vi "MarkerTactic.vi"(8 "error in (no error)":errorcluster, 9 "Game in":refnum<class "Game.lvclass">, 10 "Robot":refnum<class "Robot.lvclass">, 11 "MarkerTactic in":refnum<class "MarkerTactic.lvclass">) -> (0 "error out":errorcluster, 2 "Robot out":refnum<class "Robot.lvclass">, 3 "MarkerTactic out":refnum<class "MarkerTactic.lvclass">)   [LabVIEW 2023, in "MarkerTactic.lvclass"]
uses:
  MarkerTactic.lvclass
  Robot_class/Robot.lvclass
  Game_class/Game.lvclass
  Robot_class/tactics.ctl
  MarkerTacticStates.ctl
  Tactic_class/Tactic.lvclass/Tactic.ctl
  Game_class/Game.lvclass/Game.ctl
  Parameters_class/Parameters.lvclass/Parameters.ctl
  Skillbook_class/Skillbook.lvclass/Skillbook.ctl
  Robot_class/Robot.lvclass/Robot.ctl
  Skillbook_class/Read MarkerSkill.lvclass.vi
  Skillbook_class/Read FollowAttackerSkill.lvclass.vi
  Game_class/Read Parameters.lvclass.vi
  Parameters_class/Read Type of Marker.vi
  Parameters_class/Read DistanceStop.vi
  Tactic_class/Read Skillbook.vi
  Robot_class/Write tactic.vi
  Parameters_class/Parameters.lvclass
  Skillbook_class/Skillbook.lvclass
  MarkerSkill_class/MarkerSkill.lvclass
  FollowAttackerSkill_class/FollowAttackerSkill.lvclass
panel:
  out "x .or. y?":bool
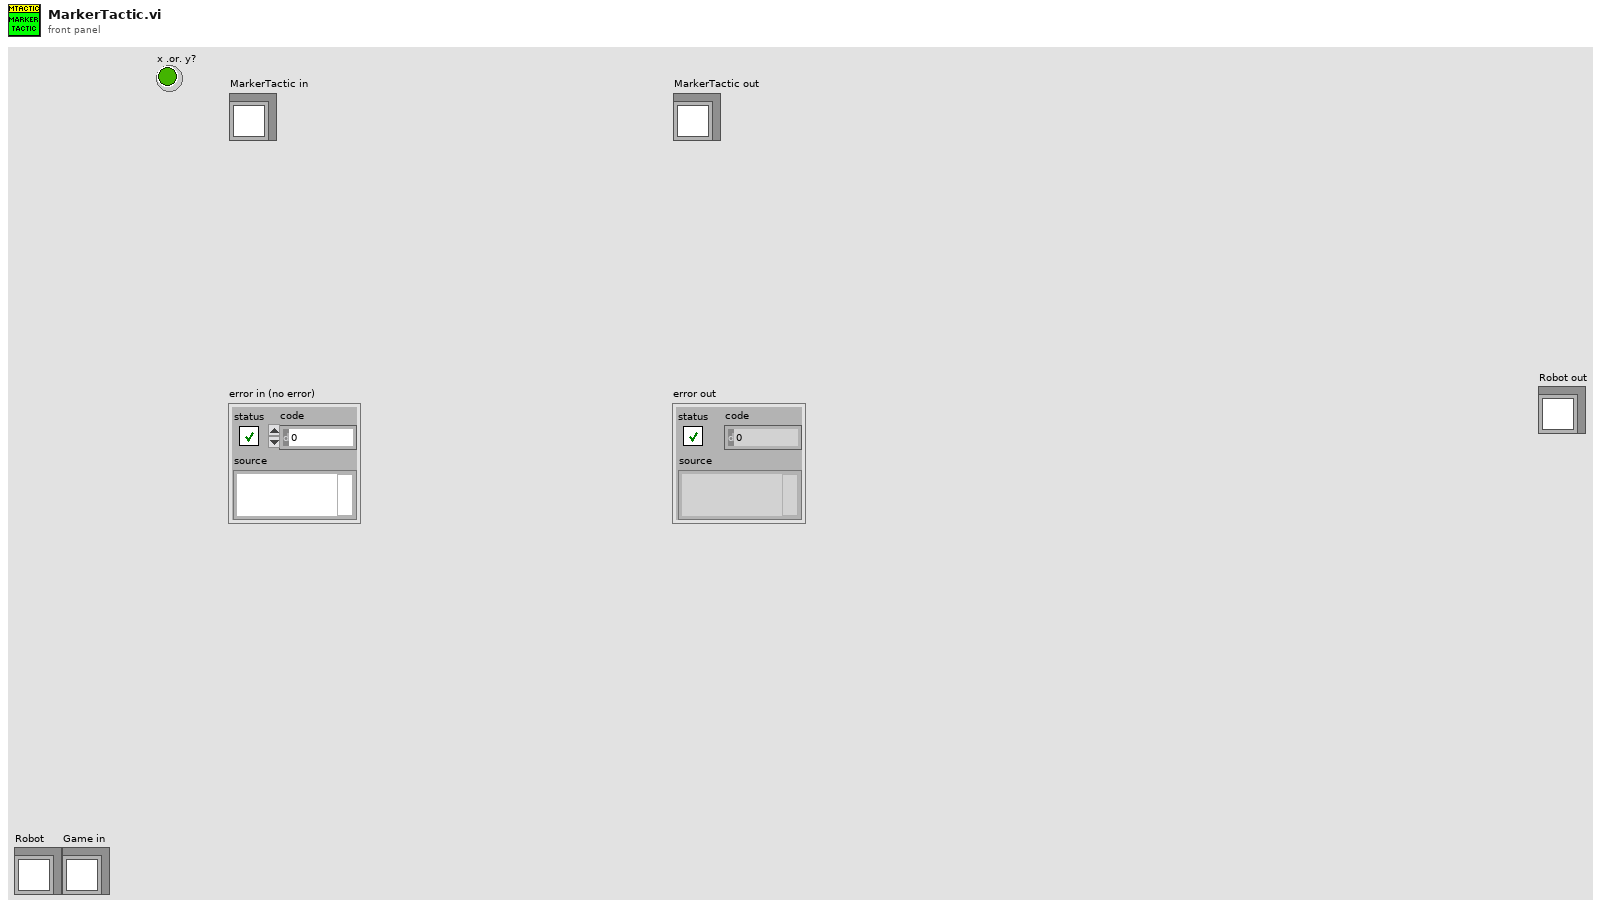
[diagram p1: front panel]
types:
  T1 = typedef "MarkerTacticStates.ctl" = enum16{"Exit", "BlockOurGoal", "FollowAttacker", "BlockEnemyPass"}
  T2 = typedef "tactics.ctl" = enum16{"ReceivePassInFuturePoint", "Roller", "PrepareRollToPassRollerGoTo", "PrepareRollToPassReceiverGoTo", "WaitRoll", "PositionToRoll", "PenaltyAttacker", "PassObserver", "PenaltyDefense", "TableReceiverTactic", "Test", "DefendGoal", "Marker", "FollowAttacker", "DefendArea", "Shoot", "AttackerAimGoal", "AttackerBallOutOfField", "AttackerBlock", "AttackerStop", "Duelist", "Halt", "ZigZag", "GoTo", "Timeout", "KickToPassReceiver", "PositionToReceivePass", "DefendAreaVSS", "DefendGoalVSS", "KickVSS", "AttackVSS", "DispBallVSS", "PenaltyAttackVSS", "WaitPass"}
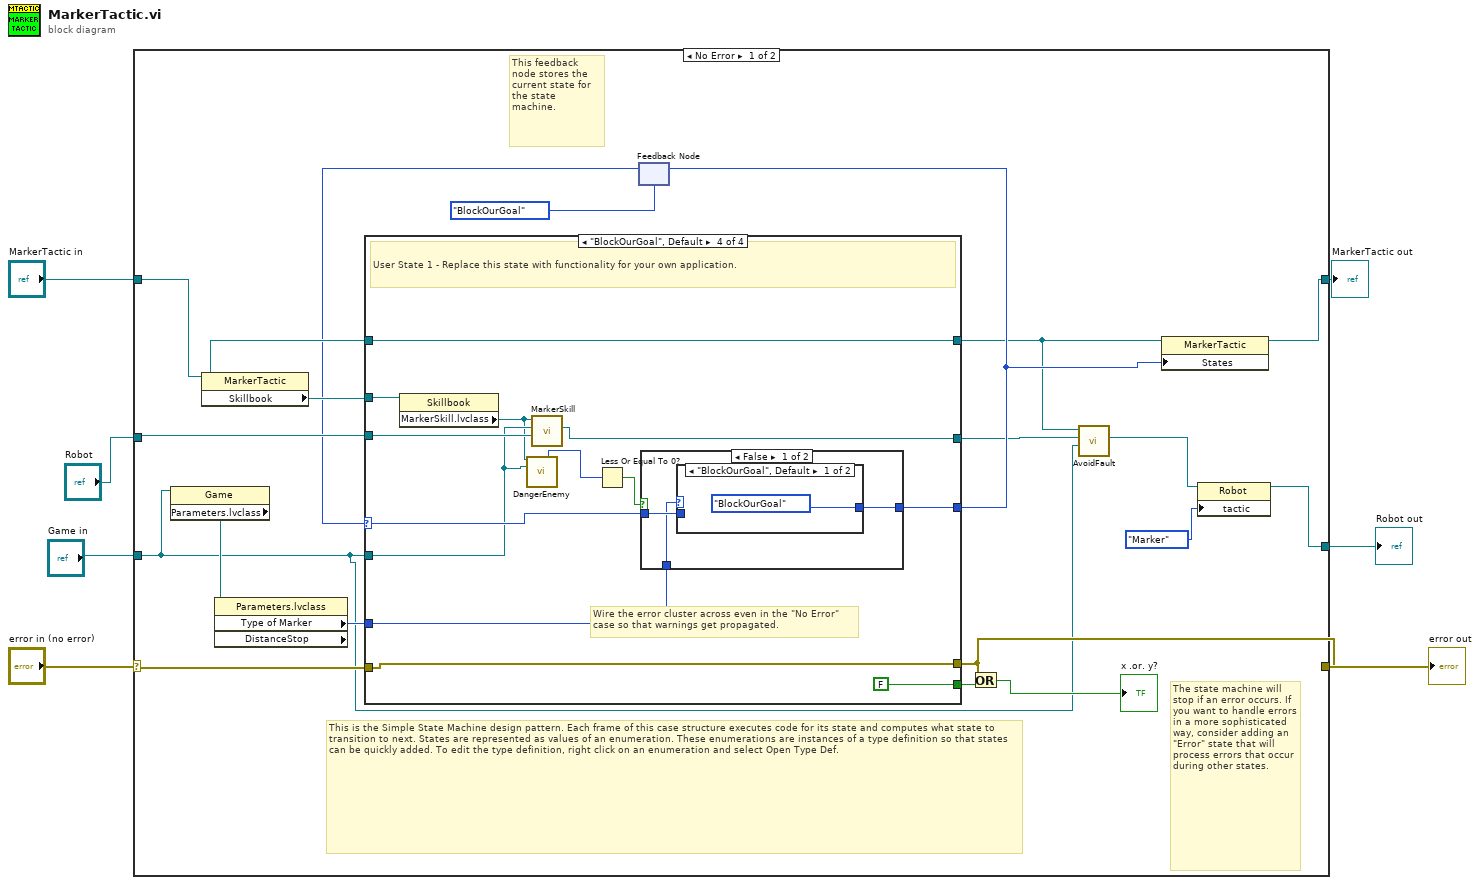
[diagram p0: block diagram]
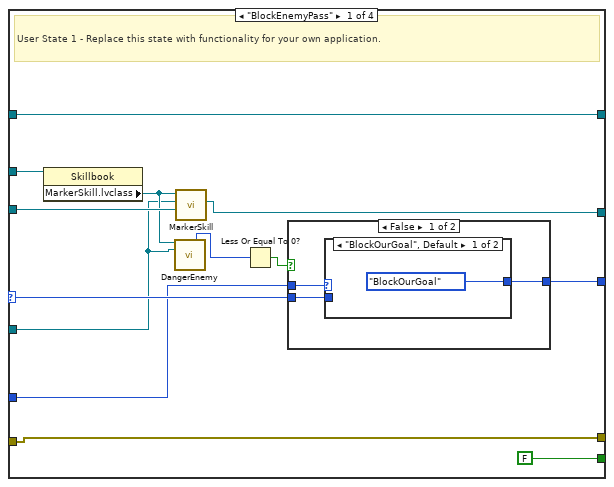
[diagram p2: hidden frame]
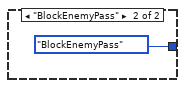
[diagram p3: hidden frame]
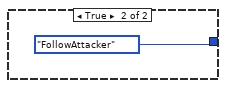
[diagram p4: hidden frame]
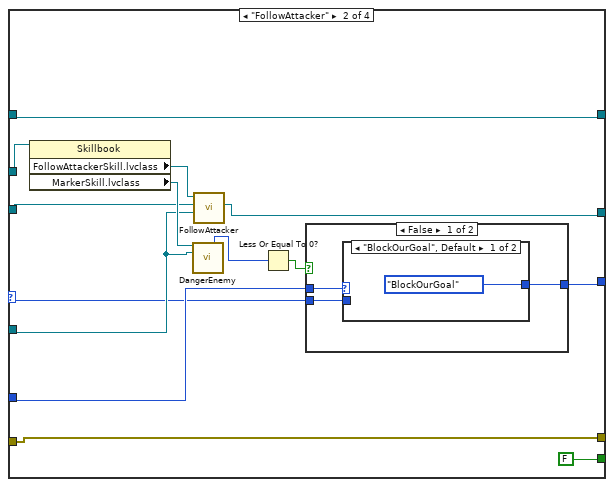
[diagram p5: hidden frame]
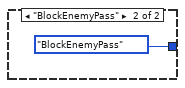
[diagram p6: hidden frame]
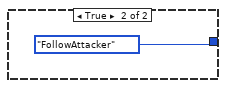
[diagram p7: hidden frame]
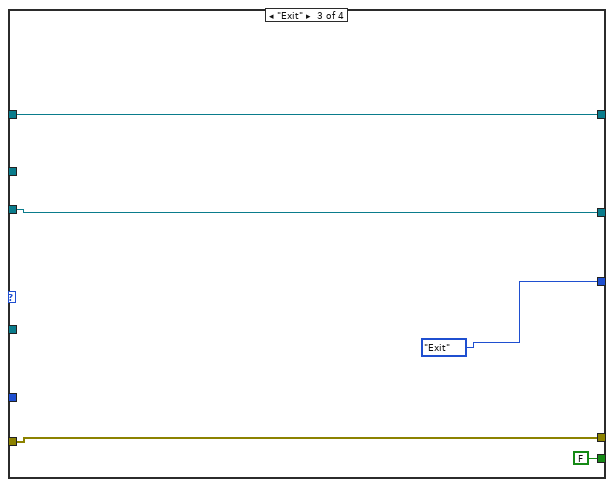
[diagram p8: hidden frame]
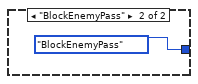
[diagram p9: hidden frame]
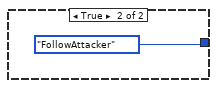
[diagram p10: hidden frame]
diagram:
  n1 = case shown="No Error" "error in (no error)" {
    selector: "error in (no error)" -> [w22 w92]
    tunnel: [w21 w92] -> w6
    tunnel: [w19 w91] -> w4
    tunnel: "MarkerTactic in" -> [w20 w91]
    tunnel: "Robot" -> [w23 w90]
    tunnel: "Game in" -> [w8 _]
    tunnel: [w14 w90] -> w1
    frame No Error {
      # "The state machine will stop if an error occurs. If you want to handle errors in a more sophisticated way, consider adding an \"Error\" state that will process errors that occur during other states."
      # "This feedback node stores the current state for the state machine."
      # "This is the Simple State Machine design pattern. Each frame of this case structure executes code for its state and computes what state to transition to next. States are represented as values of an enumeration. These enumerations are instances of a type definition so that states can be quickly added. To edit the type definition, right click on an enumeration and select Open Type Def."
      # "Wire the error cluster across even in the \"No Error\"\ncase so that warnings get propagated."
      n2 = property class="Game"(reference=w8) -> ("Parameters.lvclass"=w18:refnum<class "Parameters.lvclass">)  [unwired: 1 in, 2 out]
      n3 = property class="MarkerTactic"(reference=w20) -> ("Skillbook"=w24:refnum<class "Skillbook.lvclass">)  [unwired: 1 in, 2 out]
      n4 = property class="Parameters.lvclass" props=["Type of Marker", "DistanceStop"](reference=w18) -> ("Type of Marker"=w17:enum16{"BlockEnemyPass", "BlockOurGoal"})  [unwired: 1 in, 3 out]
      n5 = feedback #1(MarkerTacticStates."BlockOurGoal" ("States")) -> (w16:T1)
      n6 = case shown="\"BlockOurGoal\", Default" w16 {
        selector: w16 -> [w32 w49 _ w76]
        tunnel: [FALSE ("Stop Loop?") FALSE ("Stop Loop?") FALSE ("Stop Loop?") FALSE ("Stop Loop?")] -> w26
        tunnel: w24 -> [w38 w53 _ w82]
        tunnel: w23 -> [w35 w52 w69 w79]
        tunnel: [w34 w55 w69 w78] -> w11
        tunnel: [w37 w54 w70 w81] -> w9
        tunnel: w20 -> [w37 w54 w70 w81]
        tunnel: w8 -> [w28 w51 _ w74]
        tunnel: [w36 w47 w68 w80] -> w21
        tunnel: w22 -> [w36 w47 w68 w80]
        tunnel: [w33 w56 MarkerTacticStates."Exit" ("States") w77] -> w13
        tunnel: w17 -> [w31 w50 _ w75]
        frame "BlockEnemyPass" {
          # "User State 1 - Replace this state with functionality for your own application."
          n7 = property class="Skillbook"(reference=w38) -> ("MarkerSkill.lvclass"=w29:refnum<class "MarkerSkill.lvclass">)  [unwired: 1 in, 2 out]
          n8 = call-dynamic "DangerEnemy.vi"("MarkerSkill in"=w29, "Game"=w28) -> ("Numero de inimigos\npossiveis para marcar"=w27:i32)  [unwired: 6 in, 7 out]
          n9 = call-dynamic "MarkerSkill.vi"("Robot"=w35, "Game"=w28, "MarkerSkill in"=w29) -> ("Robot out"=w34:refnum<class "Robot.lvclass">)  [unwired: 6 in, 2 out]
          n10 = Less Or Equal To 0?(x=w27) -> (x <= 0?=w30:bool)
          n11 = case shown="False" w30 {
            tunnel: [w42 MarkerTacticStates."FollowAttacker" ("States")] -> w33
            tunnel: w32 -> [w41 _]
            tunnel: w31 -> [w40 _]
            frame False {
              n12 = case shown="\"BlockOurGoal\", Default" w40 {
                tunnel: [MarkerTacticStates."BlockOurGoal" ("States") MarkerTacticStates."BlockEnemyPass" ("States")] -> w42
                tunnel: w41 -> [_ _]
                frame "BlockOurGoal", Default {
                }
                frame "BlockEnemyPass" {
                }
              }
            }
            frame True {
            }
          }
        }
        frame "FollowAttacker" {
          n13 = property class="Skillbook"(reference=w53) -> ("FollowAttackerSkill.lvclass"=w48:refnum<class "FollowAttackerSkill.lvclass">, "MarkerSkill.lvclass"=w58:refnum<class "MarkerSkill.lvclass">)  [unwired: 1 in, 2 out]
          n14 = call-dynamic "DangerEnemy.vi"("MarkerSkill in"=w58, "Game"=w51) -> ("Numero de inimigos\npossiveis para marcar"=w57:i32)  [unwired: 6 in, 7 out]
          n15 = call-dynamic "FollowAttacker.vi"("Game"=w51, "Robot"=w52, "FollowAttackerSkill in"=w48) -> ("Robot out"=w55:refnum<class "Robot.lvclass">)  [unwired: 6 in, 2 out]
          n16 = Less Or Equal To 0?(x=w57) -> (x <= 0?=w59:bool)
          n17 = case shown="False" w59 {
            tunnel: [w62 MarkerTacticStates."FollowAttacker" ("States")] -> w56
            tunnel: w49 -> [w61 _]
            tunnel: w50 -> [w60 _]
            frame False {
              n18 = case shown="\"BlockOurGoal\", Default" w60 {
                tunnel: [MarkerTacticStates."BlockOurGoal" ("States") MarkerTacticStates."BlockEnemyPass" ("States")] -> w62
                tunnel: w61 -> [_ _]
                frame "BlockOurGoal", Default {
                }
                frame "BlockEnemyPass" {
                }
              }
            }
            frame True {
            }
          }
        }
        frame "Exit" {
        }
        frame "BlockOurGoal", Default {
          # "User State 1 - Replace this state with functionality for your own application."
          n19 = property class="Skillbook"(reference=w82) -> ("MarkerSkill.lvclass"=w73:refnum<class "MarkerSkill.lvclass">)  [unwired: 1 in, 2 out]
          n20 = call-dynamic "DangerEnemy.vi"("MarkerSkill in"=w73, "Game"=w74) -> ("Numero de inimigos\npossiveis para marcar"=w72:i32)  [unwired: 6 in, 7 out]
          n21 = call-dynamic "MarkerSkill.vi"("Robot"=w79, "Game"=w74, "MarkerSkill in"=w73) -> ("Robot out"=w78:refnum<class "Robot.lvclass">)  [unwired: 6 in, 2 out]
          n22 = Less Or Equal To 0?(x=w72) -> (x <= 0?=w71:bool)
          n23 = case shown="False" w71 {
            tunnel: [w86 MarkerTacticStates."FollowAttacker" ("States")] -> w77
            tunnel: w76 -> [w85 _]
            tunnel: w75 -> [w84 _]
            frame False {
              n24 = case shown="\"BlockOurGoal\", Default" w84 {
                tunnel: [MarkerTacticStates."BlockOurGoal" ("States") MarkerTacticStates."BlockEnemyPass" ("States")] -> w86
                tunnel: w85 -> [_ _]
                frame "BlockOurGoal", Default {
                }
                frame "BlockEnemyPass" {
                }
              }
            }
            frame True {
            }
          }
        }
      }
      n25 = feedback-in #1(w13) -> ()
      n26 = Or(x=w21, y=w26) -> (x .or. y?=→"x .or. y?":bool)
      n27 = call "AvoidFault.vi"("Game"=w8, "Robot in"=w11, "MarkerTactic in"=w9) -> ("Robot out"=w10:refnum<class "Robot.lvclass">)  [unwired: 6 in, 2 out]
      n28 = property class="MarkerTactic"(reference=w9, "States"=w13) -> (reference out=w19:refnum<class "MarkerTactic.lvclass">)  [unwired: 1 in, 1 out]
      n29 = property class="Robot"(reference=w10, "tactic"=tactics."Marker") -> (reference out=w14:refnum<class "Robot.lvclass">)  [unwired: 1 in, 1 out]
    }
    frame Error {
    }
  }
  "error out" <- w6
  "MarkerTactic out" <- w4
  "Robot out" <- w1
